vi "GenCalcRate.vi"(8 "TIme (s)":dbl, 11 "Distance (units)":dbl) -> (0 "Rate (units/s)":dbl)   [LabVIEW 2020]
doc: "Calculate rate for general purpose\n Inputs: time in seconds, and distnce in units\nCalculates rate value (Distance/time(s))"
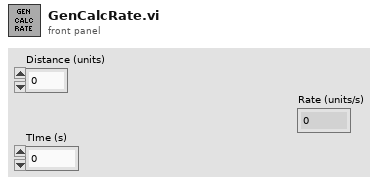
[diagram p1: front panel]
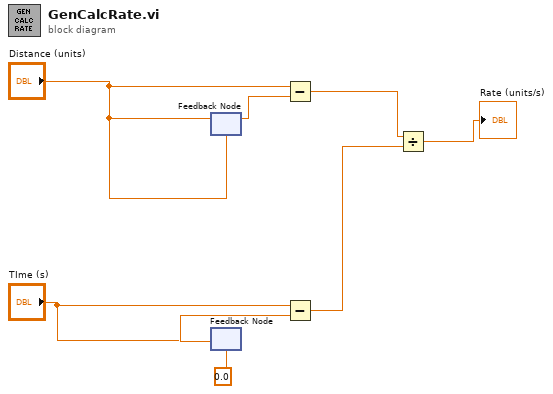
[diagram p0: block diagram]
diagram:
  n1 = feedback #1("Distance (units)") -> (w5:dbl)
  n2 = feedback-in #1("Distance (units)") -> ()
  n3 = feedback-in #2("TIme (s)") -> ()
  n4 = feedback #2(0.0 ("TIme (s)")) -> (w4:dbl)
  n5 = Subtract(x="Distance (units)", y=w5) -> (x-y=w8:dbl)
  n6 = Subtract(x="TIme (s)", y=w4) -> (x-y=w7:dbl)
  n7 = Divide(x=w8, y=w7) -> (x/y=→"Rate (units/s)":dbl)
